vi "correction_beamshaper_simu.vi"() -> ()   [LabVIEW 2020, in "ILAO_BeamShaper.lvclass"]
uses:
  ILAO_BeamShaper/ILAO_BeamShaper.lvclass
  HASO4_3/WaveKit/Controls/InteractionMatrixToCommandMatrixParameters.ctl
  HASO4_3/WaveKit/Classes/CorrectionDataManager/CorrectionDataManager.lvclass
  HASO4_3/WaveKit/Classes/Pupil/Pupil.lvclass
  HASO4_3/WaveKit/Controls/Point2Df.ctl
  HASO4_3/WaveKit/Controls/CircularPupilDetectionParams.ctl
  HASO4_3/WaveKit/Controls/PupilDetectionOption.ctl
  HASO4_3/WaveKit/Controls/CircularAutoDetectionOptions.ctl
  HASO4_3/WaveKit/Controls/PupilDetectionMode.ctl
  HASO4_3/WaveKit/Controls/WavefrontModalReconstructionType.ctl
  HASO4_3/WaveKit/Classes/ComputePhaseSet/ComputePhaseSet.lvclass
  HASO4_3/WaveKit/Controls/WavefrontReconstructionMode.ctl
  HASO4_3/WaveKit/Classes/ModalCoef/ModalCoef.lvclass
  HASO4_3/WaveKit/Controls/ZernikeModalPrefs.ctl
  HASO4_3/WaveKit/Controls/ZernikeProjectionPupilSetup.ctl
  HASO4_3/WaveKit/Classes/HasoSlopes/HasoSlopes.lvclass
panel:
  out "error out":errorcluster
  out "Delta commands":sgl[](graph)
  in  "Prefs":T1={"Number of kept modes"=32, "Tilt filtering"=FALSE}
  in  "Zernike Value":dbl[](array[numeric])=[0.0, 0.0, 0.0, 0.0, 0.0, 0.0, 0.0, 0.0, 0.0]
  in  "Normalization":bool
  in  "Interaction matrix path":path
  in  "Haso config file path":path
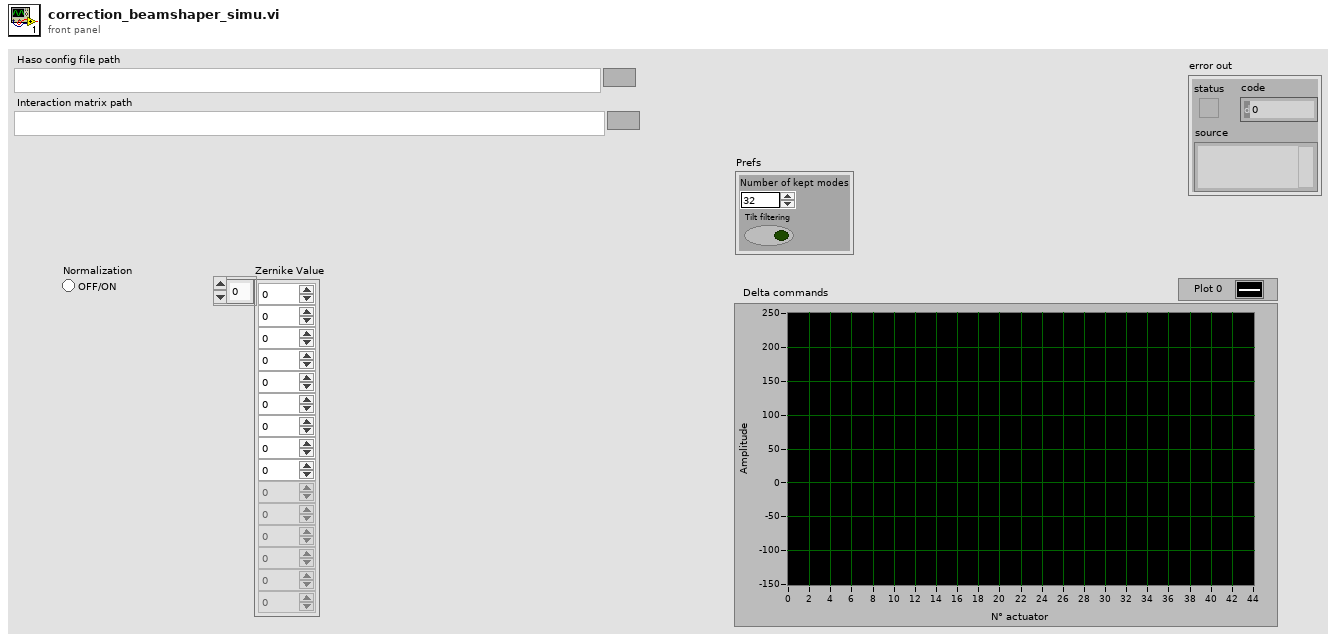
[diagram p1: front panel]
types:
  T1 = typedef "InteractionMatrixToCommandMatrixParameters.ctl" = cluster{"Number of kept modes":i32, "Tilt filtering":bool}
  T2 = typedef "ZernikeModalPrefs.ctl" = cluster{"Number of coefficients":u32, "Filtered coefficients":u32[], "RMS Zernike normalization":bool, "CircularProjectionPupilDimensions":T3}
  T3 = typedef "ZernikeProjectionPupilSetup.ctl" = cluster{"Pupil center_sspp":T4, "Pupil radius_sspp":sgl}
  T4 = typedef "Point2Df.ctl" = cluster{"X":sgl, "Y":sgl}
  T5 = typedef "WavefrontReconstructionMode.ctl" = enum16{"None", "Modal_Legendre", "Modal_Zernike", "Zonal", "Modal_Zonal_Zernike", "Modal_Zonal_Legendre"}
  T6 = typedef "WavefrontModalReconstructionType.ctl" = enum16{"Legendre", "Zernike"}
  T7 = typedef "CircularPupilDetectionParams.ctl" = cluster{"PupilDetectionOption":T8, "AutoDetectionOption":T9, "PupilDetectionMode":T10, "CentralOccultationDetection":bool}
  T8 = typedef "PupilDetectionOption.ctl" = enum16{"Manual", "Automatic"}
  T9 = typedef "CircularAutoDetectionOptions.ctl" = enum16{"manual_radius_auto_center", "manual_center_auto_radius", "auto_radius_auto_center"}
  T10 = typedef "PupilDetectionMode.ctl" = enum16{"inscribed", "circumscribed"}
  T11 = typedef "CasaoManagerGeneralSpecifications.ctl" = cluster{"Wavefront corrector name":string, "Wavefront corrector serial number":string, "Nb actuators":i32, "HASO serial number":string, "Dimension_um":T12}
  T12 = typedef "General dimensions definition.ctl" = cluster{"Size":T13, "Step":T4}
  T13 = typedef "Point2D.ctl" = cluster{"X":u32, "Y":u32}
  T14 = typedef "Wavefront Corrector Position.ctl" = sgl[]
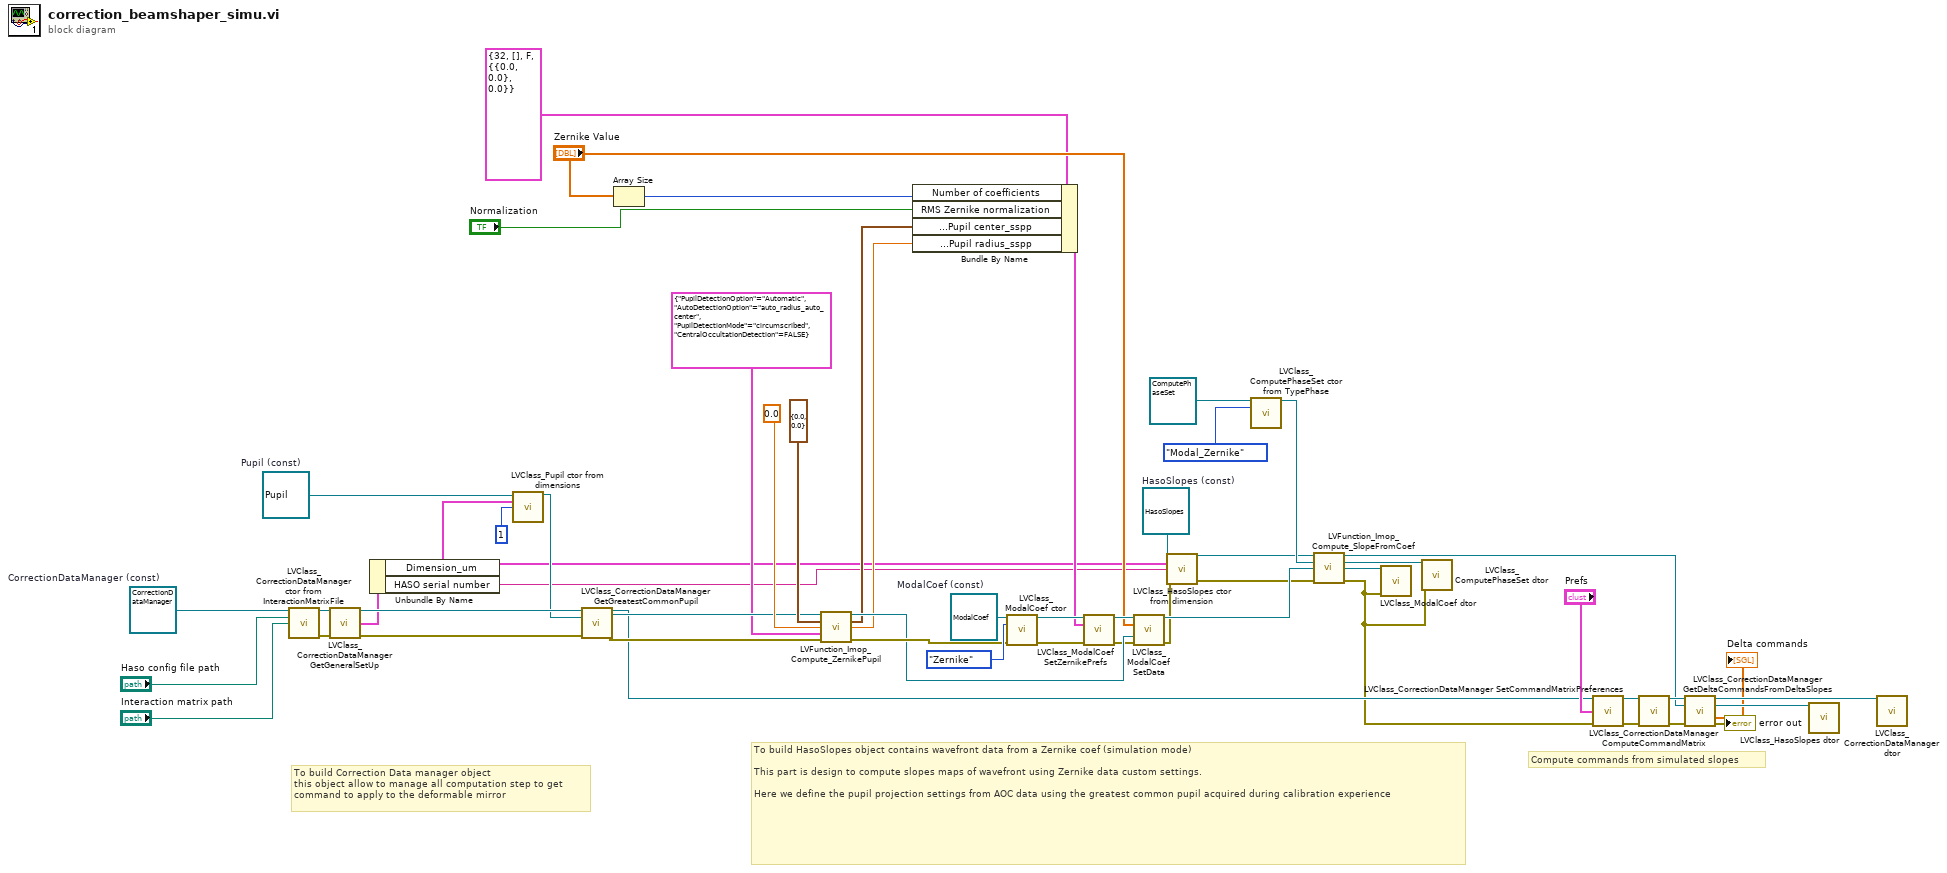
[diagram p0: block diagram]
diagram:
  w16 = refnum<class "HasoSlopes.lvclass"> refnum  # HasoSlopes (const)
  w40 = refnum<class "ModalCoef.lvclass"> refnum  # ModalCoef (const)
  w49 = refnum<class "Pupil.lvclass"> refnum  # Pupil (const)
  w48 = refnum<class "CorrectionDataManager.lvclass"> refnum  # CorrectionDataManager (const)
  # "Compute commands from simulated slopes"
  # "To build HasoSlopes object contains wavefront data from a Zernike coef (simulation mode)\n\nThis part is design to compute slopes maps of wavefront using Zernike data custom settings.\n\nHere we define the pupil projection settings from AOC data using the greatest common pupil acquired during calibration experience"
  # "To build Correction Data manager object\nthis object allow to manage all computation step to get \ncommand to apply to the deformable mirror"
  n1 = call "LVClass_CorrectionDataManager ctor from InteractionMatrixFile.vi"("CorrectionDataManager (const)"=w48, "Haso config file path"="Haso config file path", "Interaction matrix path"="Interaction matrix path") -> ("CorrectionDataManager (new)"=w55:refnum<class "CorrectionDataManager.lvclass">, "error out"=w51:errorcluster)  [unwired: 11 in]
  n2 = call "LVClass_CorrectionDataManager GetGeneralSetUp.vi"("CorrectionDataManager in"=w55, "error in (no error)"=w51) -> ("CorrectionDataManager out"=w54:refnum<class "CorrectionDataManager.lvclass">, "general"=w27:T11, "error out"=w50:errorcluster)  [unwired: 11 in]
  n3 = Unbundle By Name(w27) -> ("Dimension_um"=w15:T12, "HASO serial number"=w1:string)
  n4 = call "LVClass_Pupil ctor from dimensions.vi"("Pupil (const)"=w49, "Dimensions_um"=w15, "value"=u8 1) -> ("Pupil (new)"=w52:refnum<class "Pupil.lvclass">)  [unwired: 11 in, 1 out]
  n5 = call "LVClass_CorrectionDataManager GetGreatestCommonPupil.vi"("CorrectionDataManager in"=w54, "Pupil in"=w52, "error in (no error)"=w50) -> ("CorrectionDataManager out"=w8:refnum<class "CorrectionDataManager.lvclass">, "Pupil out"=w43:refnum<class "Pupil.lvclass">, "error out"=w41:errorcluster)  [unwired: 10 in]
  n6 = Array Size(array="Zernike Value") -> (size(s)=w22:i32)
  n7 = call "LVFunction_Imop_Compute_ZernikePupil.vi"("Pupil.lvclass"=w43, "center in"=T4 {"X"=0.0, "Y"=0.0}, "radius in"=sgl 0.0, "CircularPupilDetectionParams"=T7 {"PupilDetectionOption"=enum."Automatic", "AutoDetectionOption"=enum."auto_radius_auto_center", "PupilDetectionMode"=enum."circumscribed", "CentralOccultationDetection"=FALSE}, "error in"=w41) -> ("Pupil.lvclass"=w25:refnum<class "Pupil.lvclass">, "center"=w18:T4, "radius"=w17:sgl, "error out"=w26:errorcluster)  [unwired: 7 in]
  n8 = Bundle By Name(cluster=T2 {"Number of coefficients"=32, "Filtered coefficients"=[], "RMS Zernike normalization"=FALSE, "CircularProjectionPupilDimensions"={"Pupil center_sspp"={"X"=0.0, "Y"=0.0}, "Pupil radius_sspp"=0.0}} ("ZernikeModalPrefs 2"), "Number of coefficients"=w22, "RMS Zernike normalization"="Normalization", "CircularProjectionPupilDimensions.Pupil center_sspp"=w18, "CircularProjectionPupilDimensions.Pupil radius_sspp"=w17) -> (w20:T2)
  n9 = call "LVClass_ModalCoef ctor.vi"("ModalCoef (const)"=w40, "TypePhase"=WavefrontModalReconstructionType."Zernike", "error in (no error)"=w26) -> ("ModalCoef (new)"=w38:refnum<class "ModalCoef.lvclass">, "error out"=w39:errorcluster)  [unwired: 11 in]
  n10 = call "LVClass_ModalCoef SetZernikePrefs.vi"("ModalCoef in"=w38, "ZernikeModalPrefs"=w20, "error in (no error)"=w39) -> ("ModalCoef out"=w37:refnum<class "ModalCoef.lvclass">, "error out"=w24:errorcluster)  [unwired: 11 in]
  n11 = call "LVClass_ModalCoef SetData.vi"("ModalCoef in"=w37, "coef"="Zernike Value", "Pupil.lvclass"=w25, "error in (no error)"=w24) -> ("ModalCoef out"=w31:refnum<class "ModalCoef.lvclass">, "error out"=w29:errorcluster)  [unwired: 8 in, 2 out]
  n12 = call "LVClass_HasoSlopes ctor from dimension.vi"("HasoSlopes (const)"=w16, "Dimensions_um"=w15, "serial"=w1, "error in (no error)"=w29) -> ("HasoSlopes (new)"=w28:refnum<class "HasoSlopes.lvclass">, "error out"=w14:errorcluster)  [unwired: 10 in]
  n13 = call "LVClass_ComputePhaseSet ctor from TypePhase.vi"("ComputePhaseSet (const)"=refnum<class "ComputePhaseSet.lvclass"> refnum ("ComputePhaseSet"), "TypePhase"=WavefrontReconstructionMode."Modal_Zernike") -> ("ComputePhaseSet (new)"=w30:refnum<class "ComputePhaseSet.lvclass">)  [unwired: 12 in, 1 out]
  n14 = call "LVFunction_Imop_Compute_SlopeFromCoef.vi"("HasoSlopes.lvclass"=w28, "ComputePhaseSet"=w30, "ModalCoef.lvclass"=w31, "error IO"=w14) -> ("HasoSlopes.lvclass"=w7:refnum<class "HasoSlopes.lvclass">, "ComputePhaseSet (dup)"=w32:refnum<class "ComputePhaseSet.lvclass">, "ModalCoef.lvclass (dup)"=w33:refnum<class "ModalCoef.lvclass">, "error IO out"=w6:errorcluster)  [unwired: 8 in]
  n15 = call "LVClass_ModalCoef dtor.vi"("ModalCoef in"=w33, "error in (no error)"=w6) -> ()  [unwired: 12 in, 2 out]
  n16 = call "LVClass_ComputePhaseSet dtor.vi"("ComputePhaseSet in"=w32, "error in (no error)"=w6) -> ()  [unwired: 12 in, 2 out]
  n17 = call "LVClass_CorrectionDataManager SetCommandMatrixPreferences.vi"("CorrectionDataManager in"=w8, "Prefs"="Prefs", "error in (no error)"=w6) -> ("CorrectionDataManager out"=w12:refnum<class "CorrectionDataManager.lvclass">, "error out"=w13:errorcluster)  [unwired: 11 in]
  n18 = call "LVClass_CorrectionDataManager ComputeCommandMatrix.vi"("CorrectionDataManager in"=w12, "error in (no error)"=w13) -> ("CorrectionDataManager out"=w11:refnum<class "CorrectionDataManager.lvclass">, "error out"=w10:errorcluster)  [unwired: 12 in]
  n19 = call "LVClass_CorrectionDataManager GetDeltaCommandsFromDeltaSlopes.vi"("CorrectionDataManager in"=w11, "Delta Slopes IN"=w7, "error in (no error)"=w10) -> ("CorrectionDataManager out"=w4:refnum<class "CorrectionDataManager.lvclass">, "Delta Slope OUT"=w5:refnum<class "HasoSlopes.lvclass">, "DeltaPosition"=→"Delta commands":T14, "error out"=→"error out":errorcluster)  [unwired: 9 in]
  n20 = call "LVClass_HasoSlopes dtor.vi"("HasoSlopes in"=w5) -> ()  [unwired: 13 in, 2 out]
  n21 = call "LVClass_CorrectionDataManager dtor.vi"("CorrectionDataManager in"=w4) -> ()  [unwired: 13 in, 2 out]
